vi "Modify Yields.vi"(8 "error in (no error)":errorcluster, 10 "Boolean":bool=TRUE, 11 "Programing Logic in":refnum<class "Programing Logic.lvclass">) -> (0 "error out":errorcluster, 3 "Programing Logic out":refnum<class "Programing Logic.lvclass">)   [LabVIEW 2014, in "Programing Logic.lvclass"]
uses:
  Programing Logic.lvclass
  Programing Logic.lvclass/Programing Logic.ctl
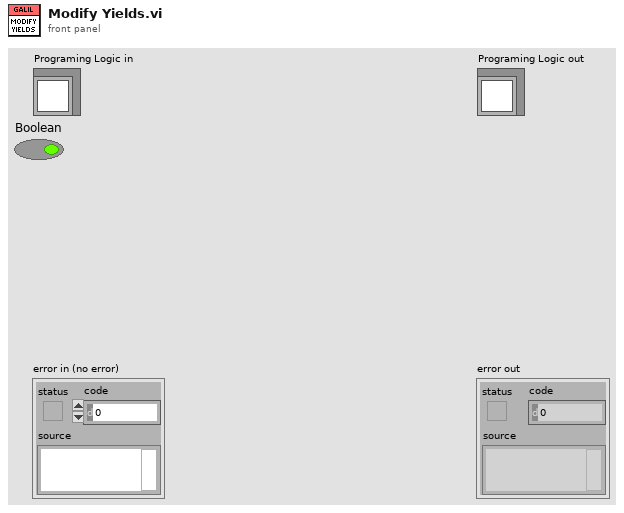
[diagram p1: front panel]
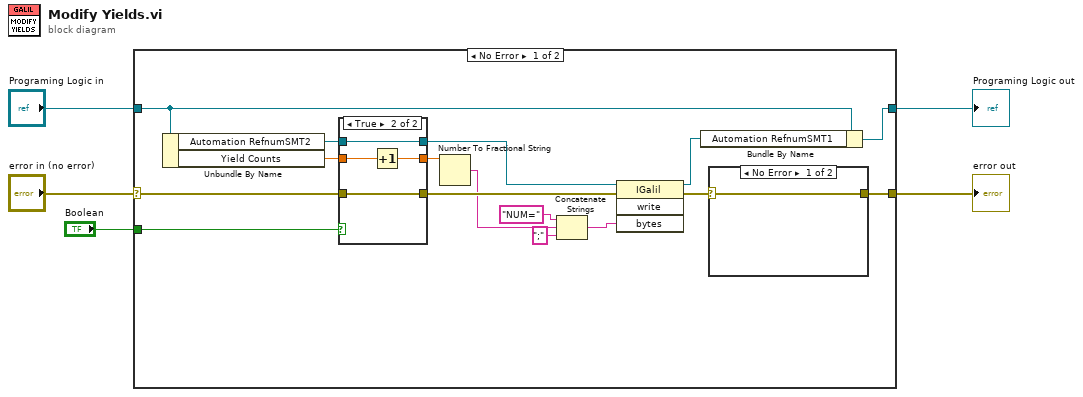
[diagram p0: block diagram]
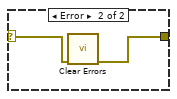
[diagram p2: hidden frame]
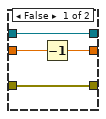
[diagram p3: hidden frame]
diagram:
  n1 = case shown="No Error" "error in (no error)" {
    selector: "error in (no error)" -> [w15 w34]
    tunnel: [w6 w34] -> w4
    tunnel: [w20 w33] -> w2
    tunnel: "Programing Logic in" -> [w21 w33]
    tunnel: "Boolean" -> [w16 _]
    frame No Error {
      n2 = Unbundle By Name(w21) -> ("Automation RefnumSMT2"=w9:refnum<k7>, "Yield Counts"=w13:dbl)
      n3 = case shown="True" w16 {
        tunnel: w15 -> [w28 w32]
        tunnel: [w28 w32] -> w14
        tunnel: w13 -> [w26 w31]
        tunnel: [w27 w30] -> w12
        tunnel: w9 -> [w25 w29]
        tunnel: [w25 w29] -> w8
        frame False {
          n4 = Decrement(x=w26) -> (x-1=w27:dbl)
        }
        frame True {
          n5 = Increment(x=w31) -> (x+1=w30:dbl)
        }
      }
      n6 = Number To Fractional String(number=w12) -> (F-format string=w11:string)  [unwired: 3 in]
      n7 = Concatenate Strings("NUM=" ("string"), w11, ";" ("string")) -> (w18:string)
      n8 = invoke class="IGalil" method="write"(reference=w8, error in=w14, "bytes"=w18) -> (reference out=w19:refnum<k7>, error out=w7:errorcluster)  [unwired: 1 in, 2 out]
      n9 = Bundle By Name(cluster=w21, "Automation RefnumSMT1"=w19) -> (w20:refnum<class "Programing Logic.lvclass">)
      n10 = case shown="No Error" w7 {
        selector: w7 -> [w22 w24]
        tunnel: [w22 w23] -> w6
        frame No Error {
        }
        frame Error {
          n11 = call <vilib>:"Clear Errors.vi"("error in (no error)"=w24) -> ("error out"=w23:errorcluster)  [unwired: 5 in, 1 out]
        }
      }
    }
    frame Error {
    }
  }
  "error out" <- w4
  "Programing Logic out" <- w2
